vi "Get Size 1D.vi"(8 "error in (no error)":errorcluster, 11 "Const_Str_1D in":refnum<class "Const_Str_1D.lvclass">) -> (0 "error out":errorcluster, 2 "Size":i32, 3 "Const_Str_1D out":refnum<class "Const_Str_1D.lvclass">)   [LabVIEW 2021, in "Const_Str_1D.lvclass"]
uses:
  Const_Str_1D.lvclass
  Const_Str_1D.lvclass/Const_Str_1D.ctl
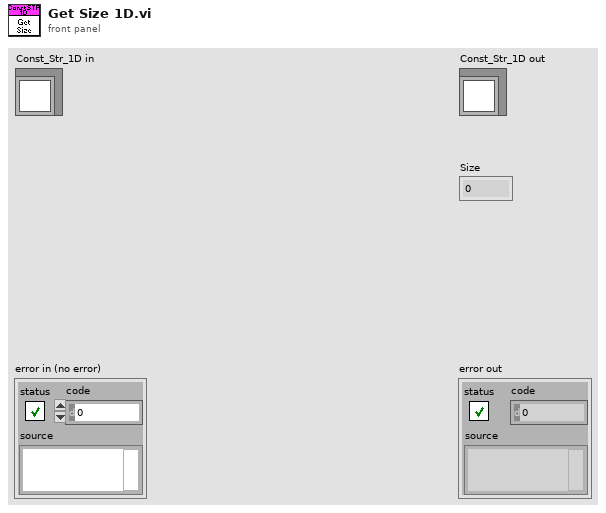
[diagram p1: front panel]
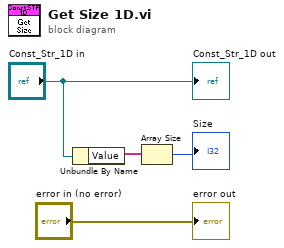
[diagram p0: block diagram]
diagram:
  n1 = Unbundle By Name("Const_Str_1D in") -> ("Value"=w3:string[])
  n2 = Array Size(array=w3) -> (size(s)=→"Size":i32)
  "error out" <- "error in (no error)"
  "Const_Str_1D out" <- "Const_Str_1D in"
